vi "Configure Setpoint Manual Track.vi"(7 "Unit Address (1)":u8=1, 8 "error in (no error)":errorcluster, 10 "Enable Manual Track  (False: Disable)":bool, 11 "VISA resource name":refnum<visa-resource-name>) -> (0 "error out":errorcluster, 3 "VISA resource name out":refnum<visa-resource-name>)   [LabVIEW 2014, in "Eurotherm 35xx Series.lvlib"]
doc: "This VI enabled or disabled Manual Track. \n\nWarning: This VI uses Controller Configuration Mode, this interrupts working process (device will not control).\nIt is recommended that the device should be disconnected from any active process."
uses:
  <instrlib>/Eurotherm 35xx Series/Eurotherm 35xx Series.lvlib
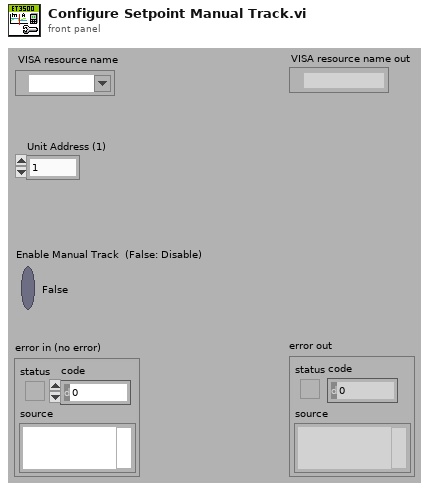
[diagram p1: front panel]
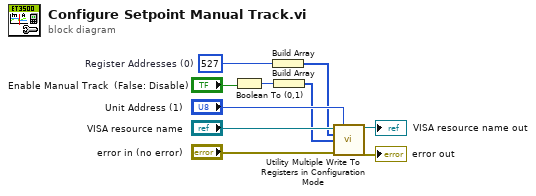
[diagram p0: block diagram]
diagram:
  w3 = 527  # Register Addresses (0)
  n1 = Boolean To (0,1)(Boolean="Enable Manual Track  (False: Disable)") -> (0, 1=w4:i16)
  n2 = Build Array(w3) -> (w1:i32[])
  n3 = Build Array(w4) -> (w2:i16[])
  n4 = call <instrlib>:"Utility Multiple Write To Registers in Configuration Mode.vi"("VISA resource name"="VISA resource name", "Unit Address (1)"="Unit Address (1)", "Registers Addresses (0)"=w1, "Data (0)"=w2, "error in (no error)"="error in (no error)") -> ("VISA resource name out"=→"VISA resource name out":refnum<visa-resource-name>, "error out"=→"error out":errorcluster)  [unwired: 9 in]
